vi "checkROIAndUpdate.vi"(5 "Settings.number of cam":dbl, 7 "Y size":i32[](array[numeric]), 9 "Settings.CamSettings 3":T1={"Cam 0"={"position"=0.0, "Field of view"=0.0, "start"=0.0, "end"=0.0, "center"=0.0, "Lens"=enum."FL1-f8x08", "Forward"=enum."off", "Spec_Calib_file 2"=path "Y:/100TWdata/ESMCalib/datFwd.txt", "map"=path "Y:/100TWdata/ESMCalib/mapFwd.txt", "y size"=0}, "Cam 1"={"position"=0.0, "Field of view"=0.0, "start"=0.0, "end"=0.0, "center"=0.0, "Lens"=enum."FL1-f8x08", "Forward"=enum."off", "Spec_Calib_file 2"=path "Y:/100TWdata/ESMCalib/datFwd.txt", "map"=path "Y:/100TWdata/ESMCalib/mapFwd.txt", "y size"=0}, "Cam 2"={"position"=0.0, "Field of view"=0.0, "start"=0.0, "end"=0.0, "center"=0.0, "Lens"=enum."FL1-f8x08", "Forward"=enum."off", "Spec_Calib_file 2"=path "Y:/100TWdata/ESMCalib/datFwd.txt", "map"=path "Y:/100TWdata/ESMCalib/mapFwd.txt", "y size"=0}, "Cam 3"={"position"=0.0, "Field of view"=0.0, "start"=0.0, "end"=0.0, "center"=0.0, "Lens"=enum."FL1-f8x08", "Forward"=enum."off", "Spec_Calib_file 2"=path "Y:/100TWdata/ESMCalib/datFwd.txt", "map"=path "Y:/100TWdata/ESMCalib/mapFwd.txt", "y size"=0}}, 10 "Clibration":T6={"cam 0"={"incident ANGLE COMPENSATION"=[], "field of view /pixel"=0.0, "dp/B [MeV/C/B]"=[], "charge compensation"=[], "Momentum [MeV/C]"=[], "B [T]"=1.0, "energyDependence Input"=[], "pixel angle (y)"=[], "dp [MeV/C/] "=[], "angle 2Dfor spectrumj"=[], "dp [MeV/C] 2D"=[], "charge compensation 2D"=[], "Screen&Camera 2"={"Screen Orientation"="Regular", "Screen angle"="Flat", "Lens"=enum."FL1-f8x08", "Calibration (mm/pix)"=1.0}, "ROI info"={"npix-X"=0, "npix-Y"=0, "Left [pix]"=0.0, "Top [pix]"=0.0}, "Y 2D full angle"=[]}, "cam 1"={"incident ANGLE COMPENSATION"=[], "field of view /pixel"=0.0, "dp/B [MeV/C/B]"=[], "charge compensation"=[], "Momentum [MeV/C]"=[], "B [T]"=1.0, "energyDependence Input"=[], "pixel angle (y)"=[], "dp [MeV/C/] "=[], "angle 2Dfor spectrumj"=[], "dp [MeV/C] 2D"=[], "charge compensation 2D"=[], "Screen&Camera 2"={"Screen Orientation"="Regular", "Screen angle"="Flat", "Lens"=enum."FL1-f8x08", "Calibration (mm/pix)"=1.0}, "ROI info"={"npix-X"=0, "npix-Y"=0, "Left [pix]"=0.0, "Top [pix]"=0.0}, "Y 2D full angle"=[]}, "cam 2"={"incident ANGLE COMPENSATION"=[], "field of view /pixel"=0.0, "dp/B [MeV/C/B]"=[], "charge compensation"=[], "Momentum [MeV/C]"=[], "B [T]"=1.0, "energyDependence Input"=[], "pixel angle (y)"=[], "dp [MeV/C/] "=[], "angle 2Dfor spectrumj"=[], "dp [MeV/C] 2D"=[], "charge compensation 2D"=[], "Screen&Camera 2"={"Screen Orientation"="Regular", "Screen angle"="Flat", "Lens"=enum."FL1-f8x08", "Calibration (mm/pix)"=1.0}, "ROI info"={"npix-X"=0, "npix-Y"=0, "Left [pix]"=0.0, "Top [pix]"=0.0}, "Y 2D full angle"=[]}, "cam 3"={"incident ANGLE COMPENSATION"=[], "field of view /pixel"=0.0, "dp/B [MeV/C/B]"=[], "charge compensation"=[], "Momentum [MeV/C]"=[], "B [T]"=1.0, "energyDependence Input"=[], "pixel angle (y)"=[], "dp [MeV/C/] "=[], "angle 2Dfor spectrumj"=[], "dp [MeV/C] 2D"=[], "charge compensation 2D"=[], "Screen&Camera 2"={"Screen Orientation"="Regular", "Screen angle"="Flat", "Lens"=enum."FL1-f8x08", "Calibration (mm/pix)"=1.0}, "ROI info"={"npix-X"=0, "npix-Y"=0, "Left [pix]"=0.0, "Top [pix]"=0.0}, "Y 2D full angle"=[]}}, 11 "ROI in":T5) -> (1 "Settings.CamSettings 2":T1={"Cam 0"={"position"=0.0, "Field of view"=0.0, "start"=0.0, "end"=0.0, "center"=0.0, "Lens"=enum."FL1-f8x08", "Forward"=enum."off", "Spec_Calib_file 2"=path "Y:/100TWdata/ESMCalib/datFwd.txt", "map"=path "Y:/100TWdata/ESMCalib/mapFwd.txt", "y size"=0}, "Cam 1"={"position"=0.0, "Field of view"=0.0, "start"=0.0, "end"=0.0, "center"=0.0, "Lens"=enum."FL1-f8x08", "Forward"=enum."off", "Spec_Calib_file 2"=path "Y:/100TWdata/ESMCalib/datFwd.txt", "map"=path "Y:/100TWdata/ESMCalib/mapFwd.txt", "y size"=0}, "Cam 2"={"position"=0.0, "Field of view"=0.0, "start"=0.0, "end"=0.0, "center"=0.0, "Lens"=enum."FL1-f8x08", "Forward"=enum."off", "Spec_Calib_file 2"=path "Y:/100TWdata/ESMCalib/datFwd.txt", "map"=path "Y:/100TWdata/ESMCalib/mapFwd.txt", "y size"=0}, "Cam 3"={"position"=0.0, "Field of view"=0.0, "start"=0.0, "end"=0.0, "center"=0.0, "Lens"=enum."FL1-f8x08", "Forward"=enum."off", "Spec_Calib_file 2"=path "Y:/100TWdata/ESMCalib/datFwd.txt", "map"=path "Y:/100TWdata/ESMCalib/mapFwd.txt", "y size"=0}}, 2 "Clibration out":cluster{"[0]":T7, "[1]":T7, "[2]":T7, "[3]":T7}={"[0]"={"incident ANGLE COMPENSATION"=[], "field of view /pixel"=0.0, "dp/B [MeV/C/B]"=[], "charge compensation"=[], "Momentum [MeV/C]"=[], "B [T]"=1.0, "energyDependence Input"=[], "pixel angle (y)"=[], "dp [MeV/C/] "=[], "angle 2Dfor spectrumj"=[], "dp [MeV/C] 2D"=[], "charge compensation 2D"=[], "Screen&Camera 2"={"Screen Orientation"="Regular", "Screen angle"="Flat", "Lens"=enum."FL1-f8x08", "Calibration (mm/pix)"=1.0}, "ROI info"={"npix-X"=0, "npix-Y"=0, "Left [pix]"=0.0, "Top [pix]"=0.0}, "Y 2D full angle"=[]}, "[1]"={"incident ANGLE COMPENSATION"=[], "field of view /pixel"=0.0, "dp/B [MeV/C/B]"=[], "charge compensation"=[], "Momentum [MeV/C]"=[], "B [T]"=1.0, "energyDependence Input"=[], "pixel angle (y)"=[], "dp [MeV/C/] "=[], "angle 2Dfor spectrumj"=[], "dp [MeV/C] 2D"=[], "charge compensation 2D"=[], "Screen&Camera 2"={"Screen Orientation"="Regular", "Screen angle"="Flat", "Lens"=enum."FL1-f8x08", "Calibration (mm/pix)"=1.0}, "ROI info"={"npix-X"=0, "npix-Y"=0, "Left [pix]"=0.0, "Top [pix]"=0.0}, "Y 2D full angle"=[]}, "[2]"={"incident ANGLE COMPENSATION"=[], "field of view /pixel"=0.0, "dp/B [MeV/C/B]"=[], "charge compensation"=[], "Momentum [MeV/C]"=[], "B [T]"=1.0, "energyDependence Input"=[], "pixel angle (y)"=[], "dp [MeV/C/] "=[], "angle 2Dfor spectrumj"=[], "dp [MeV/C] 2D"=[], "charge compensation 2D"=[], "Screen&Camera 2"={"Screen Orientation"="Regular", "Screen angle"="Flat", "Lens"=enum."FL1-f8x08", "Calibration (mm/pix)"=1.0}, "ROI info"={"npix-X"=0, "npix-Y"=0, "Left [pix]"=0.0, "Top [pix]"=0.0}, "Y 2D full angle"=[]}, "[3]"={"incident ANGLE COMPENSATION"=[], "field of view /pixel"=0.0, "dp/B [MeV/C/B]"=[], "charge compensation"=[], "Momentum [MeV/C]"=[], "B [T]"=1.0, "energyDependence Input"=[], "pixel angle (y)"=[], "dp [MeV/C/] "=[], "angle 2Dfor spectrumj"=[], "dp [MeV/C] 2D"=[], "charge compensation 2D"=[], "Screen&Camera 2"={"Screen Orientation"="Regular", "Screen angle"="Flat", "Lens"=enum."FL1-f8x08", "Calibration (mm/pix)"=1.0}, "ROI info"={"npix-X"=0, "npix-Y"=0, "Left [pix]"=0.0, "Top [pix]"=0.0}, "Y 2D full angle"=[]}}, 3 "new ROI":bool)   [LabVIEW 2011, in "MagAnalysis_Online.lvclass"]
uses:
  MagAnalysis_Online.lvclass
  calib_Sub_Typdef.ctl
  ScreenCam2_TypDEf.ctl
  CamAndObj_TypDEf.ctl
  ROIInfo_TypDef.ctl
  Calib_Typdef.ctl
  ROIStartfromCam_typdef.ctl
  CamSettings_Typdef.ctl
  CamSettingSUB_TypDEf.ctl
  OnOffTypeDef.ctl
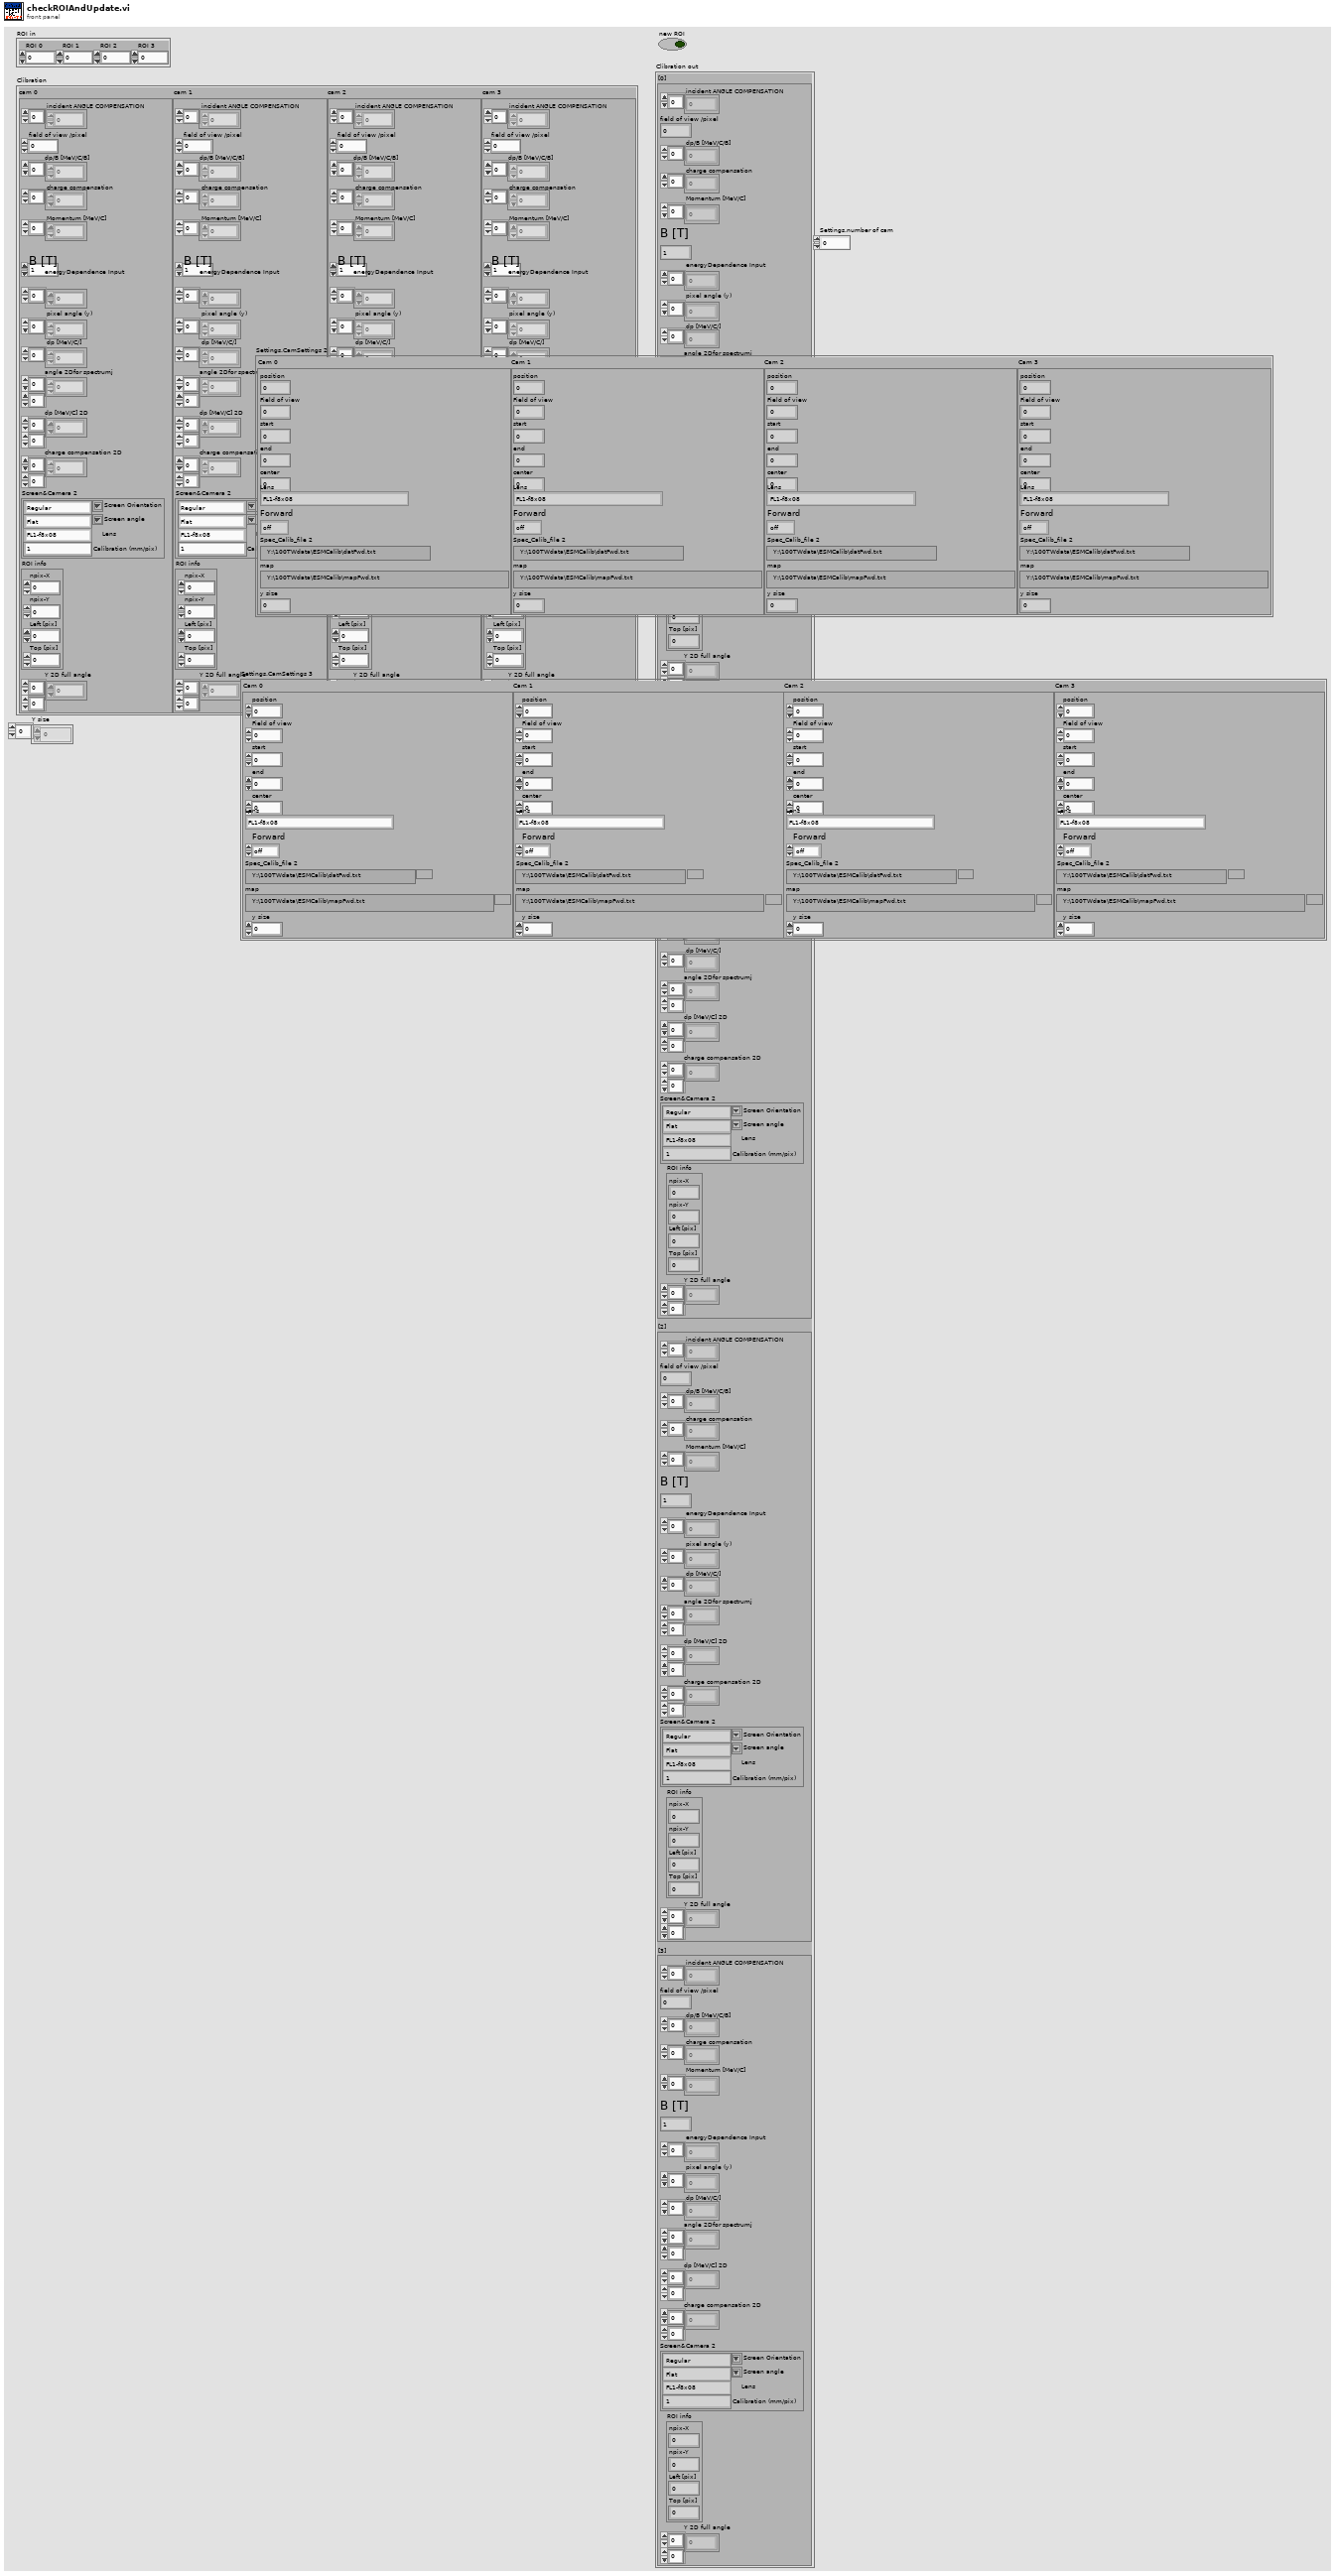
[diagram p1: front panel]
types:
  T1 = typedef "CamSettings_Typdef.ctl" = cluster{"Cam 0":T2, "Cam 1":T2, "Cam 2":T2, "Cam 3":T2}
  T2 = typedef "CamSettingSUB_TypDEf.ctl" = cluster{"position":dbl, "Field of view":dbl, "start":dbl, "end":dbl, "center":dbl, "Lens":T3, "Forward":T4, "Spec_Calib_file 2":path, "map":path, "y size":i32}
  T3 = typedef "CamAndObj_TypDEf.ctl" = enum16{"FL1-f8x08", "FL1-f8x06", "FL1-f8", "ch300-f50", "FL2G-f8", "FL3M14-f8", "FL3M14-f8x08", "FL3M14-f8x08(2x2)"}
  T4 = typedef "OnOffTypeDef.ctl" = enum16{"off", "on"}
  T5 = typedef "ROIStartfromCam_typdef.ctl" = cluster{"ROI 0":dbl, "ROI 1":dbl, "ROI 2":dbl, "ROI 3":dbl}
  T6 = typedef "Calib_Typdef.ctl" = cluster{"cam 0":T7, "cam 1":T7, "cam 2":T7, "cam 3":T7}
  T7 = typedef "calib_Sub_Typdef.ctl" = cluster{"incident ANGLE COMPENSATION":dbl[], "field of view /pixel":dbl, "dp/B [MeV/C/B]":dbl[], "charge compensation":dbl[], "Momentum [MeV/C]":dbl[], "B [T]":dbl, "energyDependence Input":dbl[], "pixel angle (y)":dbl[], "dp [MeV/C/] ":dbl[], "angle 2Dfor spectrumj":dbl[][], "dp [MeV/C] 2D":dbl[][], "charge compensation 2D":dbl[][], "Screen&Camera 2":T8, "ROI info":T9, "Y 2D full angle":dbl[][]}
  T8 = typedef "ScreenCam2_TypDEf.ctl" = cluster{"Screen Orientation":string, "Screen angle":string, "Lens":T3, "Calibration (mm/pix)":dbl}
  T9 = typedef "ROIInfo_TypDef.ctl" = cluster{"npix-X":i32, "npix-Y":i32, "Left [pix]":dbl, "Top [pix]":dbl}
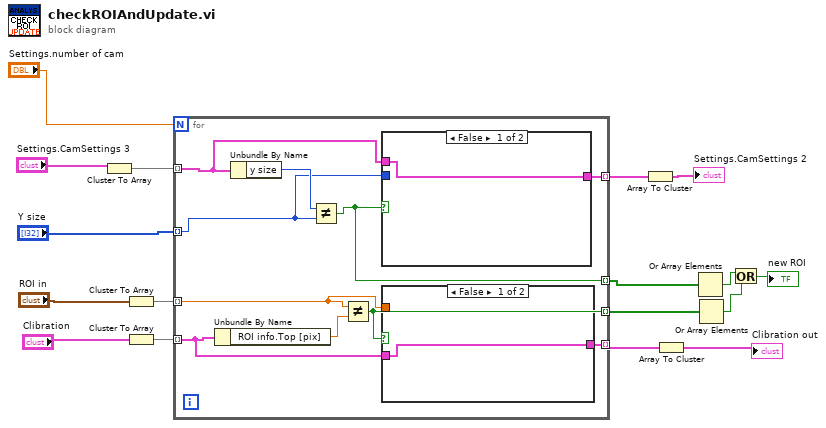
[diagram p0: block diagram]
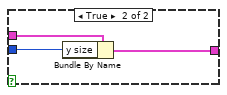
[diagram p2: hidden frame]
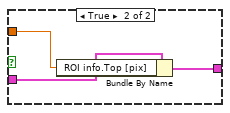
[diagram p3: hidden frame]
diagram:
  n1 = Cluster To Array(cluster="Settings.CamSettings 3") -> (array=w9:T2[])
  n2 = Cluster To Array(cluster="ROI in") -> (array=w13:dbl[])
  n3 = Cluster To Array(cluster="Clibration") -> (array=w11:T7[])
  n4 = for {
    N: "Settings.number of cam" -> [_]
    tunnel: w11 -> [w25] mode=indexing
    tunnel: w13 -> [w24] mode=indexing
    tunnel: [w26] -> w14 mode=indexing
    tunnel: [w23] -> w16 mode=indexing
    tunnel: "Y size" -> [w20] mode=indexing
    tunnel: w9 -> [w21] mode=indexing
    tunnel: [w19] -> w8 mode=indexing
    tunnel: [w18] -> w6 mode=indexing
    n5 = Unbundle By Name(w25) -> ("ROI info.Top [pix]"=w27:dbl)
    n6 = Unbundle By Name(w21) -> ("y size"=w22:i32)
    n7 = Not Equal?(x=w22, y=w20) -> (x != y?=w18:bool)
    n8 = Not Equal?(x=w24, y=w27) -> (x != y?=w26:bool)
    n9 = case shown="False" w18 {
      tunnel: w21 -> [w28 w31]
      tunnel: w20 -> [_ w30]
      tunnel: [w28 w29] -> w19
      frame False {
      }
      frame True {
        n10 = Bundle By Name(cluster=w31, "y size"=w30) -> (w29:T2)
      }
    }
    n11 = case shown="False" w26 {
      tunnel: w25 -> [w32 w35]
      tunnel: w24 -> [_ w34]
      tunnel: [w32 w33] -> w23
      frame False {
      }
      frame True {
        n12 = Bundle By Name(cluster=w35, "ROI info.Top [pix]"=w34) -> (w33:T7)
      }
    }
  }
  n13 = Array To Cluster(array=w8) -> (cluster=→"Settings.CamSettings 2":cluster{"[0]":T2, "[1]":T2, "[2]":T2, "[3]":T2})
  n14 = Array To Cluster(array=w16) -> (cluster=→"Clibration out":cluster{"[0]":T7, "[1]":T7, "[2]":T7, "[3]":T7})
  n15 = Or Array Elements(Boolean array=w6) -> (logical OR=w5:bool)
  n16 = Or Array Elements(Boolean array=w14) -> (logical OR=w4:bool)
  n17 = Or(x=w5, y=w4) -> (x .or. y?=→"new ROI":bool)
